vi "DL-Initialize Data Handling.vi"(0 "Configuration":cluster{"Stop":bool, "Config":T2}, 9 "Graph Ref":refnum<vi>, 11 "error in (no error)":errorcluster) -> (4 "file":refnum<file>, 6 ".wav":T1, 13 "path":path, 14 "frame size (s)":dbl, 15 "error out":errorcluster)   [LabVIEW 2020]
uses:
  Typedefs/DL-Configuration.ctl
  Typedefs/DL-Channel Spec.ctl
  <vilib>/sound2/lvsound2.llb/Sound File Refnum.ctl
  <vilib>/sound2/lvsound2.llb/Sound Data Format.ctl
  <vilib>/sound2/lvsound2.llb/Sound File Write Open.vi
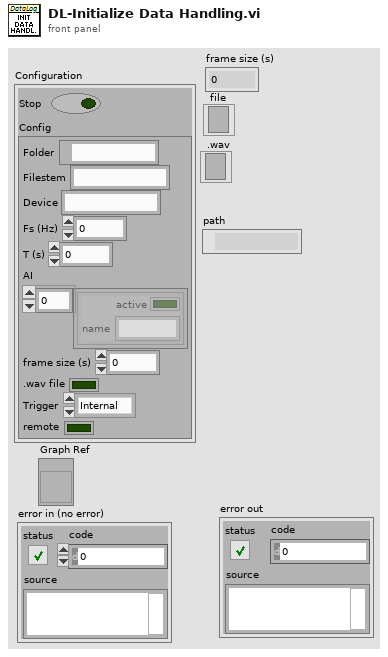
[diagram p1: front panel]
types:
  T1 = typedef "Sound File Refnum.ctl" = refnum<file>
  T2 = typedef "DL-Configuration.ctl" = cluster{"Folder":path, "Filestem":string, "Device":string, "Fs (Hz)":dbl, "T (s)":dbl, "AI":T3[], "frame size (s)":dbl, ".wav file":bool, "Trigger":enum16{"Internal", "External"}, "remote":bool}
  T3 = typedef "DL-Channel Spec.ctl" = cluster{"active":bool, "name":string}
  T4 = enum16{"open", "replace", "create", "open or create", "replace or create", "replace or create with confirmation"}
  T5 = typedef "Sound Data Format.ctl" = cluster{"sample rate (S/s)":dbl, "number of channels":i32, "bits per sample":i32}
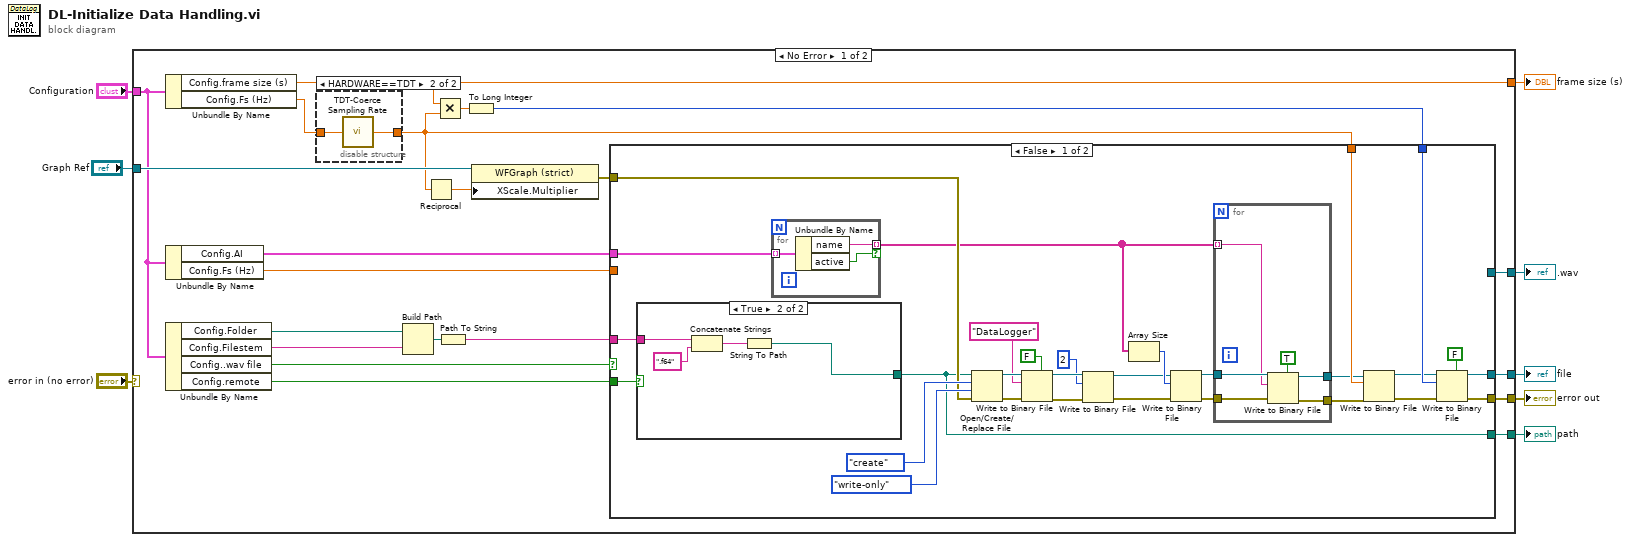
[diagram p0: block diagram]
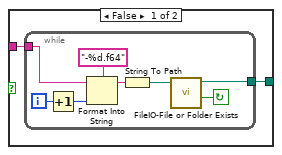
[diagram p3: hidden frame]
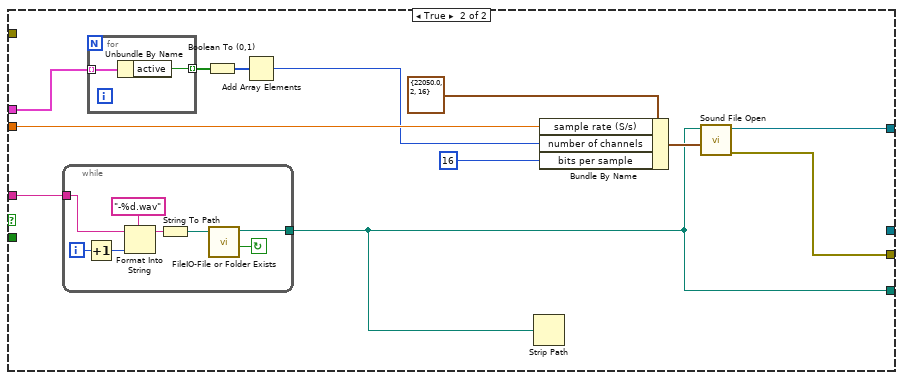
[diagram p4: hidden frame]
diagram:
  n1 = case shown="No Error" "error in (no error)" {
    selector: "error in (no error)" -> [_ w107]
    tunnel: "Configuration" -> [w22 _]
    tunnel: [w18 w107] -> w6
    tunnel: "Graph Ref" -> [w28 _]
    tunnel: [w27 _] -> w4
    tunnel: [w17 _] -> w3
    tunnel: [w13 _] -> w2
    tunnel: [w12 _] -> w1
    frame No Error {
      n2 = Unbundle By Name(w22) -> ("Config.frame size (s)"=w27:dbl, "Config.Fs (Hz)"=w10:dbl)
      n3 = Unbundle By Name(w22) -> ("Config.AI"=w21:T3[], "Config.Fs (Hz)"=w14:dbl)
      n4 = Unbundle By Name(w22) -> ("Config.Folder"=w25:path, "Config.Filestem"=w16:string, "Config..wav file"=w15:bool, "Config.remote"=w11:bool)
      n5 = disable-structure shown="HARDWARE==TDT" {
        disable-tunnel: w10 -> [w30 w32]
        disable-tunnel: [w30 w31] -> w9
        frame condition #0 {
        }
        frame condition #1 (active) {
          n6 = call "TDT-Coerce Sampling Rate.vi"("Fs (Hz)"=w32) -> ("Coerced"=w31:dbl)
        }
      }
      n7 = Build Path(base path=w25, name or relative path=w16) -> (appended path=w24:path)
      n8 = Reciprocal(x=w9) -> (1/x=w26:dbl)
      n9 = Multiply(x=w27, y=w9) -> (x*y=w29:dbl)
      n10 = Path To String(path=w24) -> (string=w23:string)
      n11 = To Long Integer(number=w29) -> (32bit integer=w19:i32)
      n12 = property class="WFGraph (strict)"(reference=w28, "XScale.Multiplier"=w26) -> (error out=w20:errorcluster)  [unwired: 1 in, 1 out]
      n13 = case shown="False" w15 {
        tunnel: w23 -> [w61 w91]
        tunnel: w21 -> [w58 w89]
        tunnel: w20 -> [w57 _]
        tunnel: w19 -> [w56 _]
        tunnel: [w54 w90] -> w18
        tunnel: [w53 _] -> w17
        tunnel: w9 -> [w50 _]
        tunnel: w14 -> [_ w93]
        tunnel: [_ w92] -> w13
        tunnel: [w44 w85] -> w12
        tunnel: w11 -> [w33 _]
        frame False {
          n14 = case shown="True" w33 {
            tunnel: w61 -> [w63 w75]
            tunnel: [w62 w72] -> w44
            frame False {
              n15 = while {
                tunnel: w63 -> [w65]
                tunnel: [w66] -> w62
                i -> [w71]
                stop <- w67 continue-if-true
                n16 = Increment(x=w71) -> (x+1=w70:i32)
                n17 = Format Into String(format string="-%d.f64", initial string=w65, w70) -> (resulting string=w69:string)  [unwired: 1 in, 1 out]
                n18 = String To Path(string=w69) -> (path=w68:path)
                n19 = call "FileIO-File or Folder Exists.vi"("path"=w68) -> ("Exists?"=w67:bool, "dup path"=w66:path)  [unwired: 7 in, 2 out]
              }
            }
            frame True {
              n20 = Concatenate Strings(w75, ".f64" ("format string")) -> (w74:string)
              n21 = String To Path(string=w74) -> (path=w72:path)
            }
          }
          n22 = for {
            tunnel: w58 -> [w84] mode=indexing
            tunnel: [w83] -> w43 mode=indexing if=w82
            n23 = Unbundle By Name(w84) -> ("name"=w83:string, "active"=w82:bool)
          }
          n24 = Open/Create/Replace File(file path (use dialog)=w44, error in=w57, operation (0:open)=T4."create", access (0:read/write)=enum16{"read/write", "read-only", "write-only"}."write-only") -> (refnum out=w41:refnum<file>, error out=w42:errorcluster)  [unwired: 2 in, 1 out]
          n25 = Write to Binary File(file (use dialog)=w41, data="DataLogger", error in=w42, 5:FALSE ("prepend array or string size? (T)")) -> (refnum out=w38:refnum<file>, error out=w35:errorcluster)  [unwired: 2 in, 1 out]
          n26 = Write to Binary File(file (use dialog)=w38, data=2, error in=w35) -> (refnum out=w37:refnum<file>, error out=w36:errorcluster)  [unwired: 3 in, 1 out]
          n27 = Array Size(array=w43) -> (size(s)=w49:i32)
          n28 = Write to Binary File(file (use dialog)=w37, data=w49, error in=w36) -> (refnum out=w46:refnum<file>, error out=w48:errorcluster)  [unwired: 3 in, 1 out]
          n29 = for {
            tunnel: w43 -> [w76] mode=indexing
            tunnel: w48 -> [w80]
            tunnel: [w79] -> w47
            tunnel: w46 -> [w78]
            tunnel: [w77] -> w45
            n30 = Write to Binary File(file (use dialog)=w78, data=w76, error in=w80, 5:TRUE ("prepend array or string size? (T)")) -> (refnum out=w77:refnum<file>, error out=w79:errorcluster)  [unwired: 2 in, 1 out]
          }
          n31 = Write to Binary File(file (use dialog)=w45, data=w50, error in=w47) -> (refnum out=w51:refnum<file>, error out=w52:errorcluster)  [unwired: 3 in, 1 out]
          n32 = Write to Binary File(file (use dialog)=w51, data=w56, error in=w52, 5:FALSE ("prepend array or string size? (T)")) -> (refnum out=w53:refnum<file>, error out=w54:errorcluster)  [unwired: 2 in, 1 out]
        }
        frame True {
          n33 = while {
            tunnel: w91 -> [w100]
            tunnel: [w101] -> w85
            i -> [w106]
            stop <- w102 continue-if-true
            n34 = Increment(x=w106) -> (x+1=w105:i32)
            n35 = Format Into String(format string="-%d.wav", initial string=w100, w105) -> (resulting string=w104:string)  [unwired: 1 in, 1 out]
            n36 = String To Path(string=w104) -> (path=w103:path)
            n37 = call "FileIO-File or Folder Exists.vi"("path"=w103) -> ("Exists?"=w102:bool, "dup path"=w101:path)  [unwired: 7 in, 2 out]
          }
          n38 = for {
            tunnel: w89 -> [w98] mode=indexing
            tunnel: [w97] -> w88 mode=indexing
            n39 = Unbundle By Name(w98) -> ("active"=w97:bool)
          }
          n40 = Boolean To (0,1)(Boolean=w88) -> (0, 1=w87:i16[])
          n41 = Add Array Elements(numeric array=w87) -> (sum=w86:i16)
          n42 = Strip Path(path=w85) -> ()  [unwired: 2 out]
          n43 = Bundle By Name(cluster=T5 {"sample rate (S/s)"=22050.0, "number of channels"=2, "bits per sample"=16} ("sound format"), "sample rate (S/s)"=w93, "number of channels"=w86, "bits per sample"=16) -> (w95:T5)
          n44 = call-poly <vilib>:"Sound File Open.vi"("sound format"=w95, "path"=w85) -> ("error out"=w90:errorcluster, "sound file refnum"=w92:T1)  [unwired: 8 in]
        }
      }
    }
    frame Error {
    }
  }
  "error out" <- w6
  "frame size (s)" <- w4
  "file" <- w3
  ".wav" <- w2
  "path" <- w1
